vi "Generate Macro Items.vi"(2 "Motion Labels":string[](array[string])=["X", "Y", "Z", "R1", "R3"], 3 "Array of TriggerAction Elements":T1[](array[typedef])) -> (0 "error out":errorcluster, 1 "Macro Items":string[][](array[string]))   [LabVIEW 2016, in "Hardware.lvlib" / "Motions.lvlib" / "Motions Configuration.lvclass"]
uses:
  <userlib>/Common Components/Hardware/Abstract System/Motions/Motions Config/Motions Configuration.lvclass
  <userlib>/Common Components/TriggerAction Q/TriggerAction Q/Element Data.ctl
  <userlib>/Common Components/Hardware/Abstract System/Motions/Motions/Data_Move.ctl
  <userlib>/Common Components/TriggerAction Q/TriggerAction Q/Trigger Cluster.ctl
  <vilib>/addons/_JKI.lib/Serialization/JSON/JKI JSON Serialization.lvlib
  <userlib>/Common Components/TriggerAction Q/TriggerAction Q/TriggerAction Q.lvclass
  <userlib>/Common Components/Hardware/Abstract System/Motions/Motions/Motions.lvclass
panel:
  out "JSON String":string
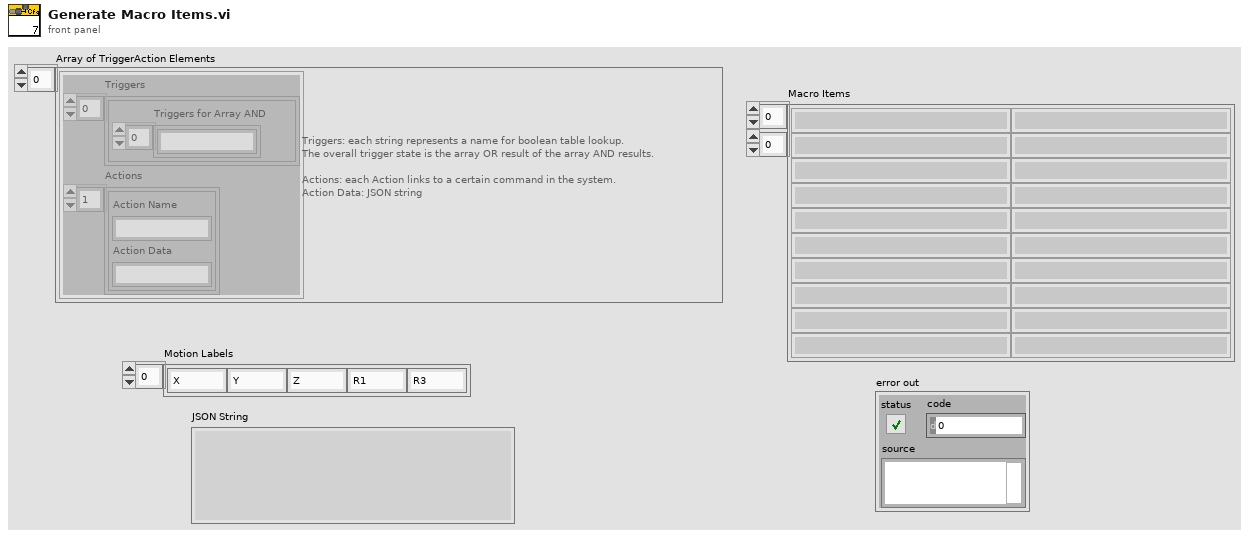
[diagram p1: front panel]
types:
  T1 = typedef "TriggerAction Q.lvclass/Element Data.ctl" = cluster{"Triggers":cluster{"Triggers for Array AND":string[]}[], "Actions":cluster{"Action Name":string, "Action Data":string}[]}
  T2 = typedef "Hardware.lvlib/Motions.lvlib/Motions.lvclass/Data_Move.ctl" = cluster{"Index":i32, "Destination":dbl}
  T3 = cluster{"Action Name":string, "Action Data":string}[]
  T4 = typedef "TriggerAction Q.lvclass/Trigger Cluster.ctl" = cluster{"Index":u8, "State Name":string}
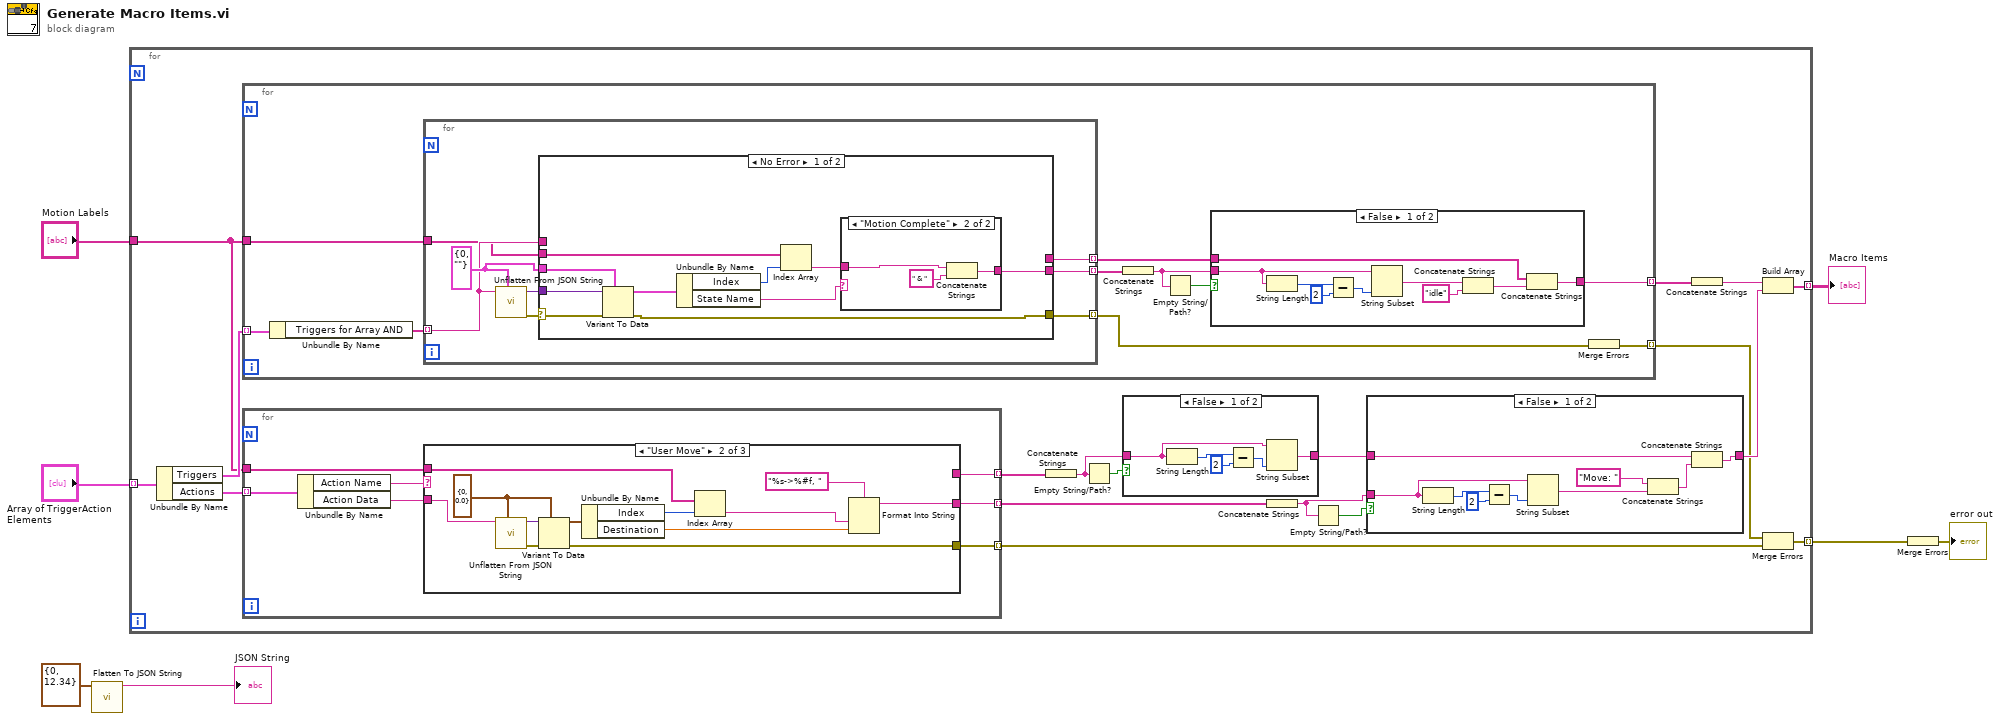
[diagram p0: block diagram]
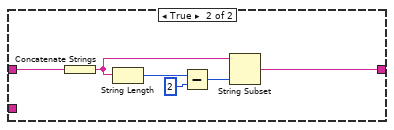
[diagram p3: hidden frame]
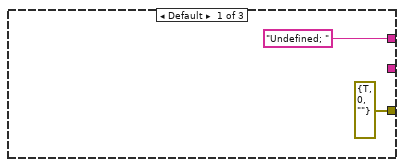
[diagram p4: hidden frame]
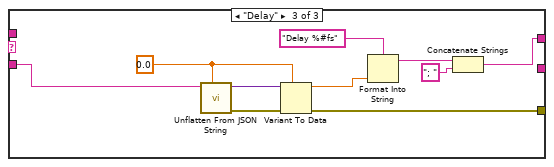
[diagram p5: hidden frame]
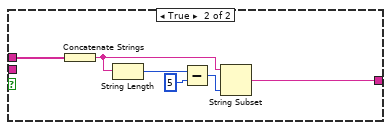
[diagram p6: hidden frame]
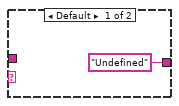
[diagram p7: hidden frame]
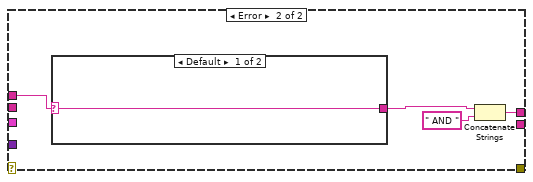
[diagram p8: hidden frame]
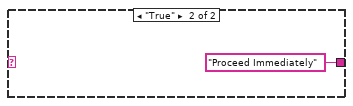
[diagram p9: hidden frame]
diagram:
  n1 = call <vilib>:"Flatten To JSON String.vi"("Variant"=T2 {"Index"=0, "Destination"=12.34} ("Move Data cluster")) -> ("JSON String"=→"JSON String":string)  [unwired: 9 in, 1 out]
  n2 = for {
    tunnel: "Array of TriggerAction Elements" -> [w25] mode=indexing
    tunnel: "Motion Labels" -> [w18]
    tunnel: [w19] -> w5 mode=indexing
    tunnel: [w13] -> w4 mode=indexing
    n3 = Unbundle By Name(w25) -> ("Triggers"=w24:cluster{"Triggers for Array AND":string[]}[], "Actions"=w22:T3)
    n4 = for {
      tunnel: w24 -> [w87] mode=indexing
      tunnel: w18 -> [w85]
      tunnel: [w82] -> w23 mode=indexing
      tunnel: [w78] -> w12 mode=indexing
      n5 = Unbundle By Name(w87) -> ("Triggers for Array AND"=w86:string[])
      n6 = for {
        tunnel: w86 -> [w108] mode=indexing
        tunnel: w85 -> [w106]
        tunnel: [w105] -> w83 mode=indexing
        tunnel: [w104] -> w84 mode=indexing
        tunnel: [w103] -> w79 mode=indexing
        w109 = T4 {"Index"=0, "State Name"=""} ("Cluster")
        n7 = call <vilib>:"Unflatten From JSON String.vi"("Type and Defaults"=w109, "JSON String"=w108) -> ("error out"=w110:errorcluster, "Variant"=w107:variant)  [unwired: 8 in]
        n8 = case shown="No Error" w110 {
          selector: w110 -> [w115 _]
          tunnel: w106 -> [w120 _]
          tunnel: w107 -> [w119 _]
          tunnel: w109 -> [w118 _]
          tunnel: [_ w125] -> w105
          tunnel: w108 -> [_ w128]
          tunnel: [w112 _] -> w104
          tunnel: [w111 _] -> w103
          frame No Error {
            n9 = Variant To Data(error in=w115, type=w118, Variant=w119) -> (data=w117:T4, error out=w111:errorcluster)
            n10 = Unbundle By Name(w117) -> ("Index"=w116:u8, "State Name"=w113:string)
            n11 = Index Array(array=w120, index=w116) -> (element=w114:string)
            n12 = case shown="\"Motion Complete\"" w113 {
              tunnel: w114 -> [_ w124]
              tunnel: ["Undefined" w122] -> w112
              frame Default {
              }
              frame "Motion Complete" {
                n13 = Concatenate Strings(w124, " & " ("string")) -> (w122:string)
              }
            }
          }
          frame Error {
            n14 = case shown="Default" w128 {
              selector: w128 -> [w129 _]
              tunnel: [w129 "Proceed Immediately"] -> w126
              frame Default {
              }
              frame "True" {
              }
            }
            n15 = Concatenate Strings(w126, " AND " ("string")) -> (w125:string)
          }
        }
      }
      n16 = Concatenate Strings(w84) -> (w81:string)
      n17 = Empty String/Path?(string/path=w81) -> (empty?=w80:bool)
      n18 = case shown="False" w80 {
        tunnel: w83 -> [w91 w98]
        tunnel: [w89 w97] -> w82
        tunnel: w81 -> [w88 _]
        frame False {
          n19 = String Length(string=w88) -> (length=w93:i32)
          n20 = Subtract(x=w93, y=2) -> (x-y=w92:i32)
          n21 = String Subset(string=w88, length (rest)=w92) -> (substring=w95:string)  [unwired: 1 in]
          n22 = Concatenate Strings(w95, "idle") -> (w90:string)
          n23 = Concatenate Strings(w91, w90) -> (w89:string)
        }
        frame True {
          n24 = Concatenate Strings(w98) -> (w99:string)
          n25 = String Length(string=w99) -> (length=w101:i32)
          n26 = Subtract(x=w101, y=5) -> (x-y=w102:i32)
          n27 = String Subset(string=w99, length (rest)=w102) -> (substring=w97:string)  [unwired: 1 in]
        }
      }
      n28 = Merge Errors(w79) -> (w78:errorcluster)
    }
    n29 = for {
      tunnel: w22 -> [w53] mode=indexing
      tunnel: [w47] -> w11 mode=indexing
      tunnel: w18 -> [w51]
      tunnel: [w49] -> w17 mode=indexing
      tunnel: [w48] -> w14 mode=indexing
      n30 = Unbundle By Name(w53) -> ("Action Name"=w52:string, "Action Data"=w50:string)
      n31 = case shown="\"User Move\"" w52 {
        tunnel: ["Undefined; " _ w68] -> w47
        tunnel: w51 -> [_ w67 _]
        tunnel: w50 -> [_ w66 w76]
        tunnel: [_ w59 _] -> w49
        tunnel: [errorcluster {"status"=TRUE, "code"=0, "source"=""} ("error out") w56 w71] -> w48
        frame Default {
        }
        frame "User Move" {
          w63 = T2 {"Index"=0, "Destination"=0.0} ("Move Data cluster")
          n32 = call <vilib>:"Unflatten From JSON String.vi"("Type and Defaults"=w63, "JSON String"=w66) -> ("error out"=w57:errorcluster, "Variant"=w64:variant)  [unwired: 8 in]
          n33 = Variant To Data(error in=w57, type=w63, Variant=w64) -> (data=w62:T2, error out=w56:errorcluster)
          n34 = Unbundle By Name(w62) -> ("Index"=w60:i32, "Destination"=w61:dbl)
          n35 = Index Array(array=w67, index=w60) -> (element=w58:string)
          n36 = Format Into String(format string="%s->%#f, " ("f"), w58, w61) -> (resulting string=w59:string)  [unwired: 2 in, 1 out]
        }
        frame "Delay" {
          w74 = 0.0
          n37 = call <vilib>:"Unflatten From JSON String.vi"("Type and Defaults"=w74, "JSON String"=w76) -> ("error out"=w72:errorcluster, "Variant"=w75:variant)  [unwired: 8 in]
          n38 = Variant To Data(error in=w72, type=w74, Variant=w75) -> (data=w73:dbl, error out=w71:errorcluster)
          n39 = Format Into String(format string="Delay %#fs", w73) -> (resulting string=w69:string)  [unwired: 2 in, 1 out]
          n40 = Concatenate Strings(w69, "; " ("string")) -> (w68:string)
        }
      }
    }
    n41 = Concatenate Strings(w11) -> (w9:string)
    n42 = Empty String/Path?(string/path=w9) -> (empty?=w10:bool)
    n43 = case shown="False" w10 {
      tunnel: w9 -> [w27 w31]
      tunnel: [w26 w31] -> w8
      frame False {
        n44 = String Length(string=w27) -> (length=w29:i32)
        n45 = Subtract(x=w29, y=2) -> (x-y=w30:i32)
        n46 = String Subset(string=w27, length (rest)=w30) -> (substring=w26:string)  [unwired: 1 in]
      }
      frame True {
      }
    }
    n47 = Concatenate Strings(w17) -> (w16:string)
    n48 = Empty String/Path?(string/path=w16) -> (empty?=w15:bool)
    n49 = case shown="False" w15 {
      tunnel: w8 -> [w40 w43]
      tunnel: [w39 w41] -> w20
      tunnel: w16 -> [w32 _]
      frame False {
        n50 = String Length(string=w32) -> (length=w37:i32)
        n51 = Subtract(x=w37, y=2) -> (x-y=w38:i32)
        n52 = String Subset(string=w32, length (rest)=w38) -> (substring=w35:string)  [unwired: 1 in]
        n53 = Concatenate Strings("Move: ", w35) -> (w33:string)
        n54 = Concatenate Strings(w40, w33) -> (w39:string)
      }
      frame True {
        n55 = Concatenate Strings(w43) -> (w42:string)
        n56 = String Length(string=w42) -> (length=w45:i32)
        n57 = Subtract(x=w45, y=2) -> (x-y=w46:i32)
        n58 = String Subset(string=w42, length (rest)=w46) -> (substring=w41:string)  [unwired: 1 in]
      }
    }
    n59 = Concatenate Strings(w23) -> (w21:string)
    n60 = Build Array(w21, w20) -> (w19:string[])
    n61 = Merge Errors(w12, w14) -> (w13:errorcluster)
  }
  "Macro Items" <- w5
  n62 = Merge Errors(w4) -> (→"error out":errorcluster)
